vi "2BLABVIEW.vi"() -> ()   [LabVIEW 2013]
panel:
  in  "INPUT":dbl
  out "OUTPUT":dbl
  in  "CONSTANT":dbl
  # "FACTORIAL OF A GIVEN NUMBER USING WHILE LOOP"
  # "N.LAKSHMI SWAPNA\n23A91A04H4"
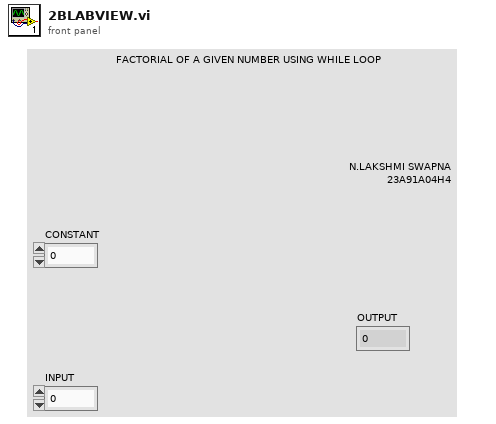
[diagram p1: front panel]
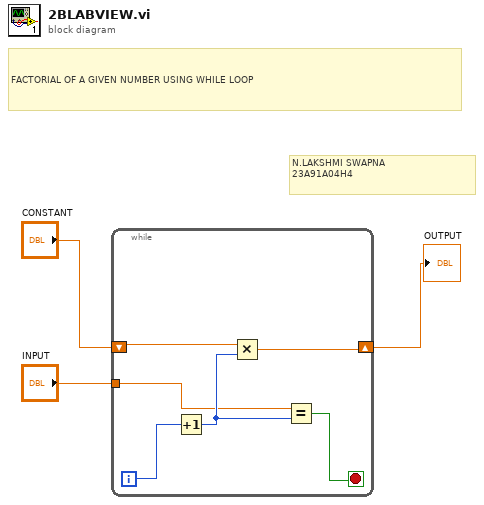
[diagram p0: block diagram]
diagram:
  # "FACTORIAL OF A GIVEN NUMBER USING WHILE LOOP"
  # "N.LAKSHMI SWAPNA\n23A91A04H4"
  n1 = while {
    shift-right: [w6] -> w3
    shift-left: "CONSTANT" -> [w5]
    tunnel: "INPUT" -> [w4]
    i -> [w9]
    stop <- w8 stop-if-true
    n2 = Increment(x=w9) -> (x+1=w7:i32)
    n3 = Multiply(x=w5, y=w7) -> (x*y=w6:dbl)
    n4 = Equal?(x=w4, y=w7) -> (x = y?=w8:bool)
  }
  "OUTPUT" <- w3
